vi "Get Timer DRV Ref.vi"(11 "TimerDRV in":refnum<class "TimerDRV.lvclass">) -> (2 "Timer DRV Ref":refnum<vi>, 3 "TimerDRV out":refnum<class "TimerDRV.lvclass">)   [LabVIEW 2019, in "TimingDRV Engine.lvlib" / "TimerDRV.lvclass"]
uses:
  TimerDRV.lvclass
  TimerDRV.lvclass/TimerDRV.ctl
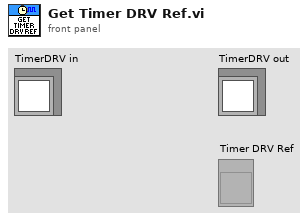
[diagram p1: front panel]
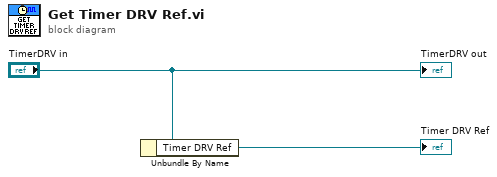
[diagram p0: block diagram]
diagram:
  n1 = Unbundle By Name("TimerDRV in") -> ("Timer DRV Ref"=→"Timer DRV Ref":refnum<vi>)
  "TimerDRV out" <- "TimerDRV in"
